vi "Build Plot.vi"(1 "Array in":dbl[][](array[numeric]), 2 "Data cluster":T1={"Time (s)"=1000.0, "Air Flow (kg/s)"=1000.0, "Air Outlet Temp (C)"=1000.0, "Air Inlet Temp (C)"=1000.0, "Sec Hot Temp (C)"=1000.0, "Sec Cold Temp (C)"=1000.0, "Sec Flow (kg/s)"=1000.0, "Pri Flow (kg/s)"=1000.0, "Pri Hot Temp (C)"=1000.0, "Pri Cold Temp (C)"=1000.0}, 3 "Boolean in":bool) -> (0 "Array out":dbl[][](array[numeric]))   [LabVIEW 2019]
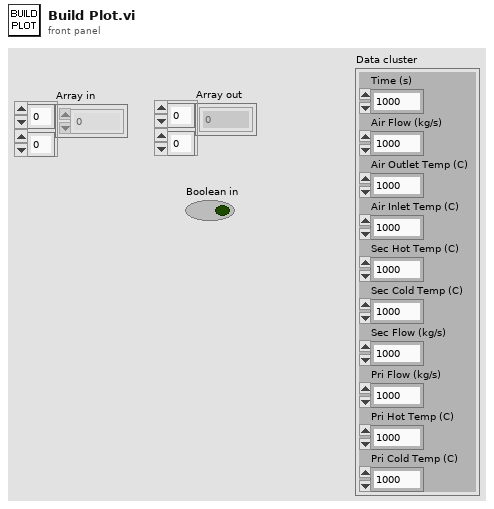
[diagram p1: front panel]
types:
  T1 = cluster{"Time (s)":dbl, "Air Flow (kg/s)":dbl, "Air Outlet Temp (C)":dbl, "Air Inlet Temp (C)":dbl, "Sec Hot Temp (C)":dbl, "Sec Cold Temp (C)":dbl, "Sec Flow (kg/s)":dbl, "Pri Flow (kg/s)":dbl, "Pri Hot Temp (C)":dbl, "Pri Cold Temp (C)":dbl}
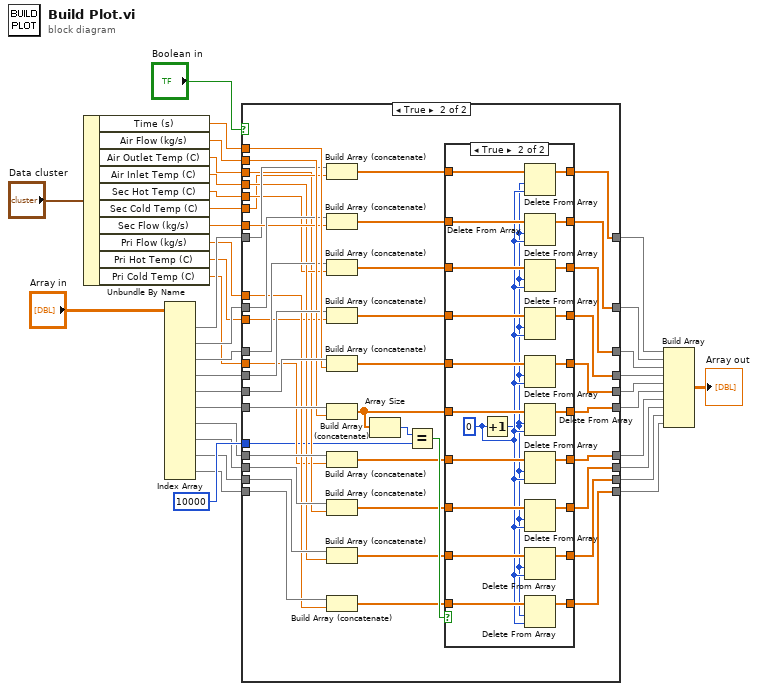
[diagram p0: block diagram]
diagram:
  n1 = Unbundle By Name("Data cluster") -> ("Time (s)"=w5:dbl, "Air Flow (kg/s)"=w4:dbl, "Air Outlet Temp (C)"=w3:dbl, "Air Inlet Temp (C)"=w2:dbl, "Sec Hot Temp (C)"=w8:dbl, "Sec Cold Temp (C)"=w10:dbl, "Sec Flow (kg/s)"=w9:dbl, "Pri Flow (kg/s)"=w1:dbl, "Pri Hot Temp (C)"=w7:dbl, "Pri Cold Temp (C)"=w6:dbl)
  n2 = Index Array(array="Array in") -> (element #1=w14:dbl[], element #2=w15:dbl[], element #3=w16:dbl[], element #4=w17:dbl[], element #5=w18:dbl[], element #6=w19:dbl[], element #7=w20:dbl[], element #8=w21:dbl[], element #9=w22:dbl[], element #10=w23:dbl[])  [unwired: 20 in]
  n3 = case shown="True" "Boolean in" {
    tunnel: w18 -> [w38 w88]
    tunnel: w5 -> [_ w87]
    tunnel: w23 -> [w37 w86]
    tunnel: w17 -> [w39 w85]
    tunnel: w20 -> [w40 w84]
    tunnel: [w39 w53] -> w29
    tunnel: [w37 w63] -> w35
    tunnel: [w38 w55] -> w30
    tunnel: w19 -> [w41 w83]
    tunnel: w4 -> [_ w82]
    tunnel: w15 -> [w44 w81]
    tunnel: w9 -> [_ w80]
    tunnel: [w41 w66] -> w31
    tunnel: [w44 w49] -> w27
    tunnel: w14 -> [w43 w79]
    tunnel: [w43 w47] -> w26
    tunnel: w16 -> [w45 w78]
    tunnel: [w45 w51] -> w28
    tunnel: [w40 w61] -> w32
    tunnel: w21 -> [w42 w77]
    tunnel: [w42 w57] -> w33
    tunnel: w22 -> [w36 w76]
    tunnel: w2 -> [_ w75]
    tunnel: [w36 w59] -> w34
    tunnel: w8 -> [_ w74]
    tunnel: w10 -> [_ w73]
    tunnel: w3 -> [_ w72]
    tunnel: w1 -> [_ w71]
    tunnel: w6 -> [_ w70]
    tunnel: w7 -> [_ w69]
    tunnel: 10000 ("x") -> [_ w46]
    frame False {
    }
    frame True {
      n4 = Build Array (concatenate)(w79, w73) -> (w48:dbl[])
      n5 = Build Array (concatenate)(w81, w80) -> (w50:dbl[])
      n6 = Build Array (concatenate)(w78, w74) -> (w52:dbl[])
      n7 = Build Array (concatenate)(w85, w69) -> (w54:dbl[])
      n8 = Build Array (concatenate)(w88, w87) -> (w56:dbl[])
      n9 = Build Array (concatenate)(w83, w82) -> (w67:dbl[])
      n10 = Build Array (concatenate)(w84, w70) -> (w62:dbl[])
      n11 = Build Array (concatenate)(w77, w72) -> (w58:dbl[])
      n12 = Build Array (concatenate)(w76, w75) -> (w60:dbl[])
      n13 = Build Array (concatenate)(w86, w71) -> (w64:dbl[])
      n14 = Array Size(array=w67) -> (size(s)=w65:i32)
      n15 = Equal?(x=w65, y=w46) -> (x = y?=w68:bool)
      n16 = case shown="True" w68 {
        tunnel: w67 -> [w98 w120]
        tunnel: [w98 w119] -> w66
        tunnel: w64 -> [w94 w118]
        tunnel: [w94 w117] -> w63
        tunnel: w62 -> [w95 w116]
        tunnel: [w95 w115] -> w61
        tunnel: w60 -> [w96 w114]
        tunnel: [w96 w113] -> w59
        tunnel: w58 -> [w97 w112]
        tunnel: [w97 w111] -> w57
        tunnel: w56 -> [w89 w110]
        tunnel: [w89 w109] -> w55
        tunnel: w54 -> [w90 w108]
        tunnel: [w90 w107] -> w53
        tunnel: w52 -> [w91 w106]
        tunnel: [w91 w105] -> w51
        tunnel: w50 -> [w92 w104]
        tunnel: [w92 w103] -> w49
        tunnel: w48 -> [w93 w100]
        tunnel: [w93 w99] -> w47
        frame False {
        }
        frame True {
          w102 = 0 ("index")
          n17 = Increment(x=w102) -> (x+1=w101:i32)
          n18 = Delete From Array(array=w100, length=w101, index=w102) -> (array with subset deleted=w99:dbl[])  [unwired: 1 out]
          n19 = Delete From Array(array=w104, length=w101, index=w102) -> (array with subset deleted=w103:dbl[])  [unwired: 1 out]
          n20 = Delete From Array(array=w106, length=w101, index=w102) -> (array with subset deleted=w105:dbl[])  [unwired: 1 out]
          n21 = Delete From Array(array=w108, length=w101, index=w102) -> (array with subset deleted=w107:dbl[])  [unwired: 1 out]
          n22 = Delete From Array(array=w110, length=w101, index=w102) -> (array with subset deleted=w109:dbl[])  [unwired: 1 out]
          n23 = Delete From Array(array=w120, length=w101, index=w102) -> (array with subset deleted=w119:dbl[])  [unwired: 1 out]
          n24 = Delete From Array(array=w116, length=w101, index=w102) -> (array with subset deleted=w115:dbl[])  [unwired: 1 out]
          n25 = Delete From Array(array=w112, length=w101, index=w102) -> (array with subset deleted=w111:dbl[])  [unwired: 1 out]
          n26 = Delete From Array(array=w114, length=w101, index=w102) -> (array with subset deleted=w113:dbl[])  [unwired: 1 out]
          n27 = Delete From Array(array=w118, length=w101, index=w102) -> (array with subset deleted=w117:dbl[])  [unwired: 1 out]
        }
      }
    }
  }
  n28 = Build Array(w26, w27, w28, w29, w30, w31, w32, w33, w34, w35) -> (→"Array out":dbl[][])
